vi "_Update Parameter Data.vi"(4 "error in":errorcluster, 7 "Parameter":T1 {"Expt"."Mass Range"."Resolution Type" items=["High/High", "Medium/Medium", "Low/Low", "High/Medium", "High/Low", "Medium/High", "Medium/Low", "Low/High", "Low/Medium"]}) -> (0 "error out":errorcluster, 3 "RF Only":bool)   [LabVIEW 2012]
uses:
  Type/_RT Parameter.ctl
  Type/_RT Active Ch.ctl
  Type/_RT Expt.ctl
  Type/_Run Mode.ctl
  Type/_RT Mass Range.ctl
  Type/_RT Res Type.ctl
  _RT Global.vi
  <vilib>/Utility/error.llb/Error Cluster From Error Code.vi
  <vilib>/rvi/errors/niLvFpgaAdjustHostInterfaceError.vi
  <vilib>/rvi/interface/nirviReadWriteControl/nirviReadWriteControl.xnode
  FPGA Bitfiles/FPGA9602.lvbitx
  NiFpgaLv.dll
panel:
  out "x-y":u32
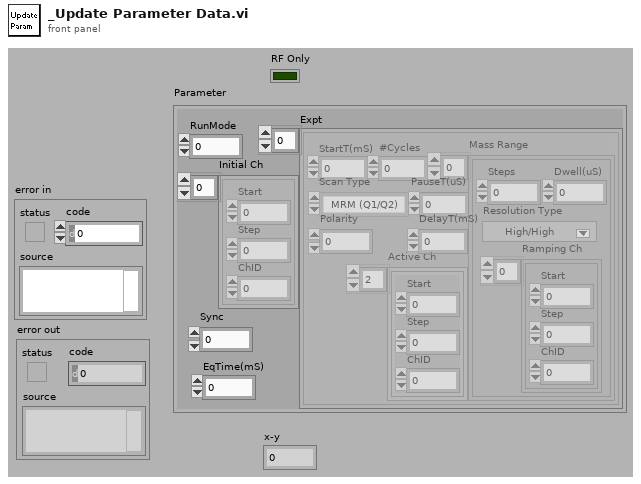
[diagram p1: front panel]
types:
  T1 = typedef "_RT Parameter.ctl" = cluster{"RunMode":i32, "Initial Ch":T2[], "Sync":u8, "Expt":T3[], "EqTime(mS)":i32}
  T2 = typedef "_RT Active Ch.ctl" = cluster{"Start":i32, "Step":i32, "ChID":i32}
  T3 = typedef "_RT Expt.ctl" = cluster{"StartT(mS)":i32, "#Cycles":i32, "Scan Type":T4, "PauseT(uS)":i32, "Polarity":u8, "DelayT(mS)":i32, "Active Ch":T2[], "Mass Range":T5[]}
  T4 = typedef "_Run Mode.ctl" = enum16{"MRM (Q1/Q2)", "Q1 Scan", "Q1 SRM", "Q2 Scan", "Q2 SRM", "Product Scan", "Precursor Scan", "Neutral Loss", "Neutral Gain"}
  T5 = typedef "_RT Mass Range.ctl" = cluster{"Steps":i32, "Dwell(uS)":i32, "Resolution Type":T6, "Ramping Ch":T2[]}
  T6 = typedef "_RT Res Type.ctl" = u16
  T7 = typedef "_RT Instrument 2.ctl" = cluster{"Table":T8[], "Instrument":string[]}
  T8 = typedef "_RT Configuration 2.ctl" = cluster{"Name":string, "Ch#":u8, "Min":dbl, "Max":dbl, "Def+":dbl, "Def-":dbl, "Offset":dbl, "Slope":dbl, "Type":u8, "Description":string, "SettleT":dbl}
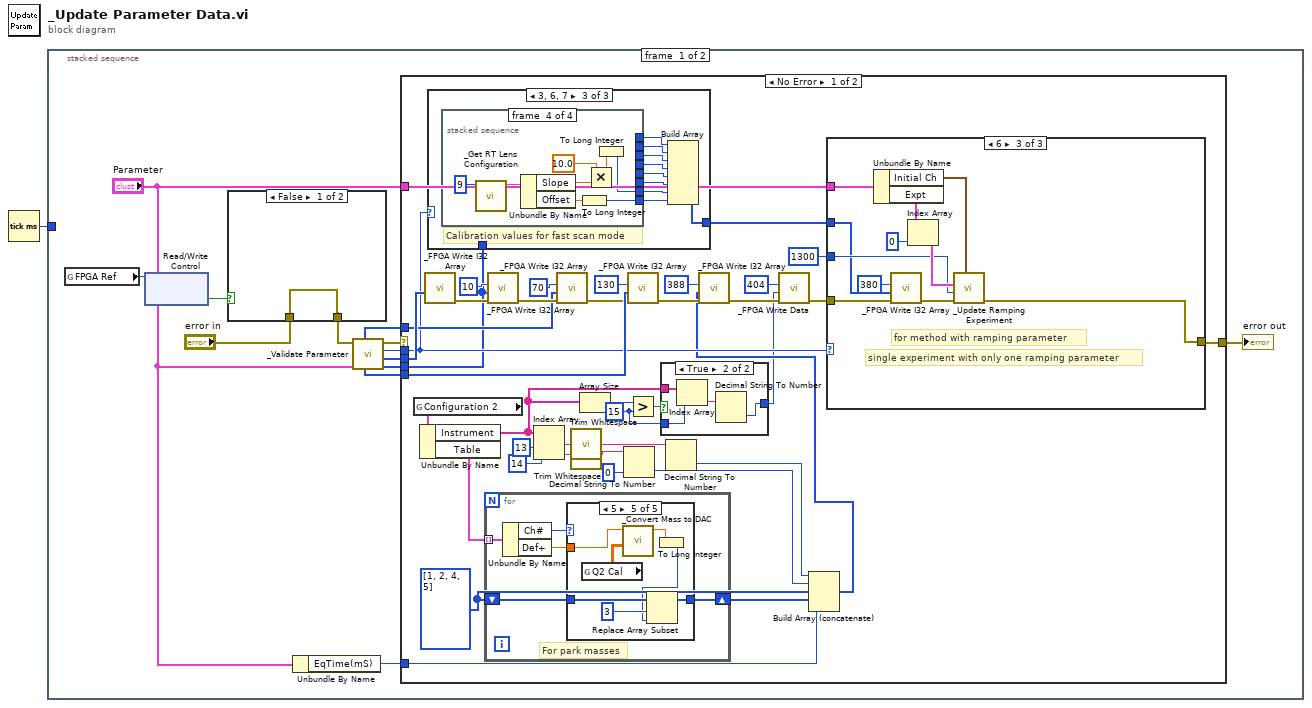
[diagram p0: block diagram]
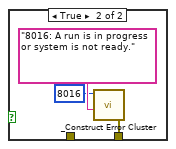
[diagram p2: hidden frame]
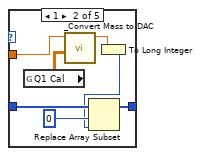
[diagram p5: hidden frame]
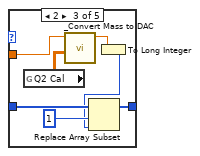
[diagram p6: hidden frame]
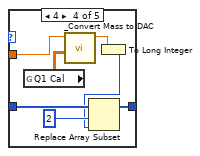
[diagram p7: hidden frame]
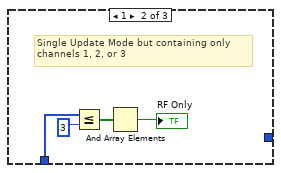
[diagram p9: hidden frame]
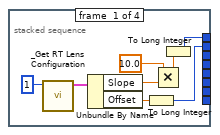
[diagram p10: hidden frame]
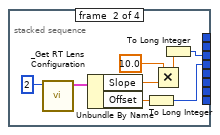
[diagram p11: hidden frame]
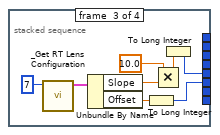
[diagram p12: hidden frame]
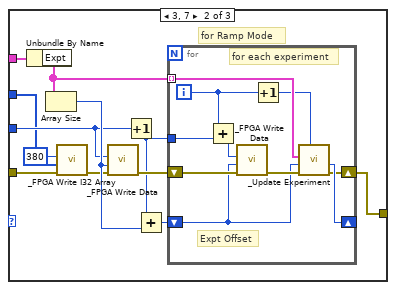
[diagram p14: hidden frame]
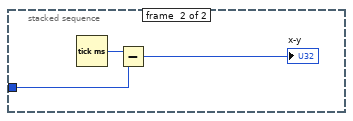
[diagram p16: hidden frame]
diagram:
  n1 = Tick Count (ms)() -> (millisecond timer value=w1:u32)
  n2 = stacked-sequence {
    tunnel: w1 -> [_ w179]
    frame #0 {
      n3 = global read "_RT Global.vi" "FPGA Ref"() -> (w2:refnum<k20>)
      n4 = xnode "Read/Write Control"("FPGA VI Reference In"=w2) -> ("Running"=w5:bool)  [unwired: 1 in, 2 out]
      n5 = case shown="False" w5 {
        tunnel: [w15 w16] -> w4
        tunnel: "error in" -> [w15 _]
        frame False {
        }
        frame True {
          n6 = call "_Construct Error Cluster.vi"("reason"="8016: A run is in progress or system is not ready.", "errorCode"=8016) -> ("error out"=w16:errorcluster)  [unwired: 2 in, 3 out]
        }
      }
      n7 = Unbundle By Name("Parameter") -> ("EqTime(mS)"=w6:i32)
      n8 = call "_Validate Parameter.vi"("Parameter"="Parameter", "error in (no error)"=w4) -> ("Ch ID"=w10:i32[], "General Param"=w11:i32[], "RunMode"=w12:i32, "error out"=w13:errorcluster, "Low Values"=w8:i32[], "High Values (DAC)"=w9:i32[])  [unwired: 2 out]
      n9 = case shown="No Error" w13 {
        selector: w13 -> [_ w177]
        tunnel: [w58 w177] -> w14
        tunnel: w12 -> [w46 _]
        tunnel: w11 -> [w56 _]
        tunnel: w10 -> [w27 _]
        tunnel: w9 -> [w51 _]
        tunnel: w8 -> [w49 _]
        tunnel: "Parameter" -> [w57 _]
        tunnel: w6 -> [w30 _]
        frame No Error {
          w20 = 15 ("y")
          w32 = i32[] [1, 2, 4, 5]
          n10 = global read "_RT Global.vi" "Configuration 2"() -> (w44:T7)
          n11 = Unbundle By Name(w44) -> ("Instrument"=w21:string[], "Table"=w37:T8[])
          n12 = call "_FPGA Write I32 Array.vi"("I32 Array"=w56) -> ("error out"=w54:errorcluster)  [unwired: 4 in, 2 out]
          n13 = case shown="3, 6, 7" w46 {
            tunnel: [_ _ w102] -> w45
            tunnel: w27 -> [_ w101 _]
            frame 0, Default {
            }
            frame 1 {
              # "Single Update Mode but containing only\nchannels 1, 2, or 3"
              n14 = Less Or Equal?(x=w101, y=3) -> (x <= y?=w99:bool[])
              n15 = And Array Elements(Boolean array=w99) -> (logical AND=→"RF Only":bool)
            }
            frame 3, 6, 7 {
              # "Calibration values for fast scan mode"
              n16 = stacked-sequence {
                tunnel: [w112 _ _ _] -> w103
                tunnel: [w111 _ _ _] -> w104
                tunnel: [_ w120 _ _] -> w105
                tunnel: [_ w119 _ _] -> w106
                tunnel: [_ _ w128 _] -> w107
                tunnel: [_ _ w127 _] -> w108
                tunnel: [_ _ _ w136] -> w109
                tunnel: [_ _ _ w135] -> w110
                frame #0 {
                  n17 = call "_Get RT Lens Configuration.vi"("Channel #"=u8 1) -> ("Lens Configuration"=w117:T8)  [unwired: 1 in, 5 out]
                  n18 = Unbundle By Name(w117) -> ("Slope"=w115:dbl, "Offset"=w116:dbl)
                  n19 = To Long Integer(number=w116) -> (32bit integer=w111:i32)
                  n20 = Multiply(x=10.0, y=w115) -> (x*y=w113:dbl)
                  n21 = To Long Integer(number=w113) -> (32bit integer=w112:i32)
                }
                frame #1 {
                  n22 = call "_Get RT Lens Configuration.vi"("Channel #"=u8 2) -> ("Lens Configuration"=w125:T8)  [unwired: 1 in, 5 out]
                  n23 = Unbundle By Name(w125) -> ("Slope"=w123:dbl, "Offset"=w124:dbl)
                  n24 = To Long Integer(number=w124) -> (32bit integer=w119:i32)
                  n25 = Multiply(x=10.0, y=w123) -> (x*y=w121:dbl)
                  n26 = To Long Integer(number=w121) -> (32bit integer=w120:i32)
                }
                frame #2 {
                  n27 = call "_Get RT Lens Configuration.vi"("Channel #"=u8 7) -> ("Lens Configuration"=w133:T8)  [unwired: 1 in, 5 out]
                  n28 = Unbundle By Name(w133) -> ("Slope"=w131:dbl, "Offset"=w132:dbl)
                  n29 = To Long Integer(number=w132) -> (32bit integer=w127:i32)
                  n30 = Multiply(x=10.0, y=w131) -> (x*y=w129:dbl)
                  n31 = To Long Integer(number=w129) -> (32bit integer=w128:i32)
                }
                frame #3 {
                  n32 = call "_Get RT Lens Configuration.vi"("Channel #"=u8 9) -> ("Lens Configuration"=w141:T8)  [unwired: 1 in, 5 out]
                  n33 = Unbundle By Name(w141) -> ("Slope"=w139:dbl, "Offset"=w140:dbl)
                  n34 = To Long Integer(number=w140) -> (32bit integer=w135:i32)
                  n35 = Multiply(x=10.0, y=w139) -> (x*y=w137:dbl)
                  n36 = To Long Integer(number=w137) -> (32bit integer=w136:i32)
                }
              }
              n37 = Build Array(w103, w104, w105, w106, w107, w108, w109, w110) -> (w102:i32[])
            }
          }
          n38 = for {
            tunnel: w37 -> [w68] mode=indexing
            shift-right: [w65] -> w31
            shift-left: w32 -> [w66]
            # "For park masses"
            n39 = Unbundle By Name(w68) -> ("Ch#"=w67:u8, "Def+"=w64:dbl)
            n40 = case shown="5" w67 {
              tunnel: w66 -> [w69 w73 w80 w87 w94]
              tunnel: [w69 w70 w77 w84 w91] -> w65
              tunnel: w64 -> [_ w76 w83 w90 w97]
              frame 0, Default {
              }
              frame 1 {
                n41 = global read "_RT Global.vi" "Q1 Cal"() -> (w75:dbl[][])
                n42 = call "_Convert Mass to DAC.vi"("Calibration Table"=w75, "Mass"=w76) -> ("DAC Value"=w74:dbl)  [unwired: 2 in, 3 out]
                n43 = To Long Integer(number=w74) -> (32bit integer=w71:i32)
                n44 = Replace Array Subset(array=w73, new element=w71, index=0) -> (w70:i32[])
              }
              frame 2 {
                n45 = global read "_RT Global.vi" "Q2 Cal"() -> (w82:dbl[][])
                n46 = call "_Convert Mass to DAC.vi"("Calibration Table"=w82, "Mass"=w83) -> ("DAC Value"=w81:dbl)  [unwired: 2 in, 3 out]
                n47 = To Long Integer(number=w81) -> (32bit integer=w78:i32)
                n48 = Replace Array Subset(array=w80, new element=w78, index=1) -> (w77:i32[])
              }
              frame 4 {
                n49 = global read "_RT Global.vi" "Q1 Cal"() -> (w89:dbl[][])
                n50 = call "_Convert Mass to DAC.vi"("Calibration Table"=w89, "Mass"=w90) -> ("DAC Value"=w88:dbl)  [unwired: 2 in, 3 out]
                n51 = To Long Integer(number=w88) -> (32bit integer=w85:i32)
                n52 = Replace Array Subset(array=w87, new element=w85, index=2) -> (w84:i32[])
              }
              frame 5 {
                n53 = global read "_RT Global.vi" "Q2 Cal"() -> (w96:dbl[][])
                n54 = call "_Convert Mass to DAC.vi"("Calibration Table"=w96, "Mass"=w97) -> ("DAC Value"=w95:dbl)  [unwired: 2 in, 3 out]
                n55 = To Long Integer(number=w95) -> (32bit integer=w92:i32)
                n56 = Replace Array Subset(array=w94, new element=w92, index=3) -> (w91:i32[])
              }
            }
          }
          n57 = call "_FPGA Write I32 Array.vi"("error in"=w54, "I32 Array"=w27, "Offset (0)"=10 ("y")) -> ("error out"=w52:errorcluster)  [unwired: 2 in, 2 out]
          n58 = Index Array(array=w21, index #1=13 ("index"), index #2=14 ("index")) -> (element #1=w41:string, element #2=w40:string)
          n59 = call "_FPGA Write I32 Array.vi"("error in"=w52, "I32 Array"=w51, "Offset (0)"=70 ("y")) -> ("error out"=w48:errorcluster)  [unwired: 2 in, 2 out]
          n60 = call <vilib>:"Trim Whitespace.vi"("string"=w41) -> ("trimmed string"=w29:string)  [unwired: 1 in]
          n61 = call <vilib>:"Trim Whitespace.vi"("string"=w40) -> ("trimmed string"=w39:string)  [unwired: 1 in]
          n62 = Array Size(array=w21) -> (size(s)=w23:i32)
          n63 = Decimal String To Number(string=w39, default (0L)=0 ("default (0 I32)")) -> (number=w36:i32)  [unwired: 2 out]
          n64 = call "_FPGA Write I32 Array.vi"("error in"=w48, "I32 Array"=w49, "Offset (0)"=130 ("y")) -> ("error out"=w35:errorcluster)  [unwired: 2 in, 2 out]
          n65 = Greater?(x=w23, y=w20) -> (0:w22:bool)
          n66 = case shown="True" w22 {
            tunnel: w21 -> [_ w63]
            tunnel: w20 -> [w59 w61]
            tunnel: [w59 w60] -> w19
            frame False {
            }
            frame True {
              n67 = Index Array(array=w63, index=w61) -> (element=w62:string)
              n68 = Decimal String To Number(string=w62) -> (number=w60:i32)  [unwired: 3 out]
            }
          }
          n69 = Decimal String To Number(string=w29) -> (number=w28:i32)  [unwired: 3 out]
          n70 = Build Array (concatenate)(w28, w36, w32, w31, w30) -> (w33:i32[])
          n71 = call "_FPGA Write I32 Array.vi"("error in"=w35, "I32 Array"=w33, "Offset (0)"=388 ("y")) -> ("error out"=w26:errorcluster)  [unwired: 2 in, 2 out]
          n72 = call "_FPGA Write Data.vi"("error in"=w26, "Data"=w19, "Address"=404 ("y")) -> ("error out"=w25:errorcluster)  [unwired: 5 in]
          n73 = case shown="6" w46 {
            tunnel: [w143 w151 w173] -> w58
            tunnel: w57 -> [_ w150 w176]
            tunnel: w25 -> [w143 w146 w168]
            tunnel: u16 1300 ("Address") -> [_ w148 w171]
            tunnel: w45 -> [_ w144 w166]
            frame Default {
            }
            frame 3, 7 {
              # "for Ramp Mode"
              n74 = Unbundle By Name(w150) -> ("Expt"=w155:T3[])
              n75 = Array Size(array=w155) -> (size(s)=w149:i32)
              n76 = call "_FPGA Write I32 Array.vi"("error in"=w146, "I32 Array"=w144, "Offset (0)"=380 ("y")) -> ("error out"=w145:errorcluster)  [unwired: 2 in, 2 out]
              n77 = call "_FPGA Write Data.vi"("error in"=w145, "Data"=w149, "Address"=w148) -> ("error out"=w154:errorcluster)  [unwired: 3 in, 2 out]
              n78 = Increment(x=w148) -> (x+1=w152:u16)
              n79 = Add(x=w152, y=w149) -> (x+y=w153:i32)
              n80 = for {
                tunnel: w155 -> [w163] mode=indexing
                shift-right: [w158] -> w151
                shift-left: w154 -> [w165]
                tunnel: w152 -> [w164]
                shift-right: [w159] -> _
                shift-left: w153 -> [w160]
                i -> [w157]
                # "for each experiment"
                # "Expt Offset"
                n81 = Add(x=w157, y=w164) -> (x+y=w161:i32)
                n82 = call "_FPGA Write Data.vi"("error in"=w165, "Data"=w160, "Address"=w161) -> ("error out"=w162:errorcluster)  [unwired: 3 in, 2 out]
                n83 = Increment(x=w157) -> (x+1=w156:i32)
                n84 = call "_Update Experiment.vi"("Expt#"=w156, "error in"=w162, "Offset"=w160, "Expt"=w163) -> ("error out"=w158:errorcluster, "Next Offset"=w159:u16)  [unwired: 1 in, 2 out]
              }
            }
            frame 6 {
              # "single experiment with only one ramping parameter"
              # "for method with ramping parameter"
              n85 = Unbundle By Name(w176) -> ("Initial Ch"=w170:T2[], "Expt"=w175:T3[])
              n86 = call "_FPGA Write I32 Array.vi"("error in"=w168, "I32 Array"=w166, "Offset (0)"=380 ("y")) -> ("error out"=w167:errorcluster)  [unwired: 2 in, 2 out]
              n87 = Index Array(array=w175, index=0) -> (element=w172:T3)
              n88 = call "_Update Ramping Experiment.vi"("Ramping Ch"=w170, "error in"=w167, "Offset"=w171, "Expt"=w172) -> ("error out"=w173:errorcluster)  [unwired: 1 in, 3 out]
            }
          }
        }
        frame Error {
        }
      }
      "error out" <- w14
    }
    frame #1 {
      n89 = Tick Count (ms)() -> (millisecond timer value=w180:u32)
      n90 = Subtract(x=w180, y=w179) -> (x-y=→"x-y":u32)
    }
  }
